vi "0-Read MDF.vi"(2 "Error in":errorcluster, 3 "MDF file path":path) -> (0 "Error out":errorcluster, 1 "Waypoints List":T1)   [LabVIEW 2011]
doc: "Reads a MDF (Mission Definition File) as saved by 0-Save MDF.vi"
uses:
  0x2-OCU-Think Comm/0x2 Typedefs/Waypoints List.ctl
  0x2-OCU-Think Comm/0x2 Typedefs/ocuWaypoint.ctl
  0x2-OCU-Think Comm/0x2 Typedefs/waypointTypes.ctl
  2-Think/2 Typedefs/UTM Location.ctl
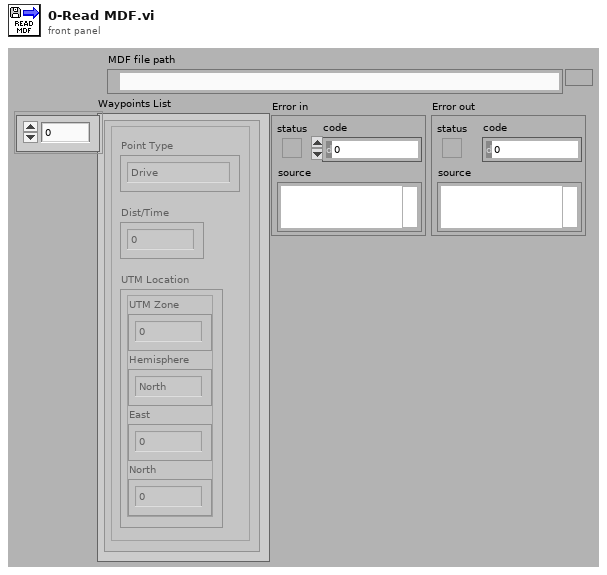
[diagram p1: front panel]
types:
  T1 = typedef "Waypoints List.ctl" = T2[]
  T2 = typedef "ocuWaypoint.ctl" = cluster{"Point Type":T3, "Dist/Time":dbl, "UTM Location":T4}
  T3 = typedef "waypointTypes.ctl" = enum16{"Drive", "Round Port", "Round Starboard", "Stay"}
  T4 = typedef "UTM Location.ctl" = cluster{"UTM Zone":dbl, "Hemisphere":enum16{"North", "South"}, "East":dbl, "North":dbl}
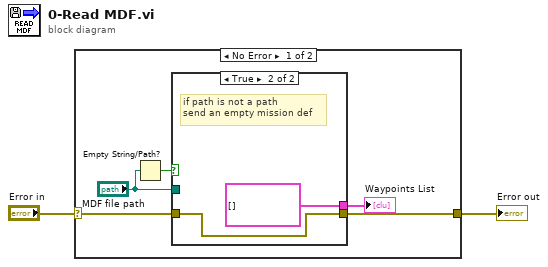
[diagram p0: block diagram]
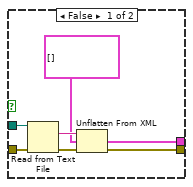
[diagram p2: hidden frame]
diagram:
  n1 = case shown="No Error" "Error in" {
    selector: "Error in" -> [w4 w17]
    tunnel: [w3 w17] -> w1
    frame No Error {
      n2 = Empty String/Path?(string/path="MDF file path") -> (empty?=w7:bool)
      n3 = case shown="True" w7 {
        tunnel: [w10 T1 [] ("Waypoints List 2")] -> w5
        tunnel: "MDF file path" -> [w14 _]
        tunnel: w4 -> [w9 w15]
        tunnel: [w8 w15] -> w3
        frame False {
          n4 = Read from Text File(file (use dialog)=w14, error in=w9) -> (text=w13:string, error out=w12:errorcluster)  [unwired: 2 in, 2 out]
          n5 = Unflatten From XML(xml string=w13, type=T1 [] ("Waypoints List 2"), error in (no error)=w12) -> (value=w10:T1, error out=w8:errorcluster)
        }
        frame True {
          # "if path is not a path\nsend an empty mission def"
        }
      }
      "Waypoints List" <- w5
    }
    frame Error {
    }
  }
  "Error out" <- w1
